vi "Main.vi"(11 "Module Admin":refnum<class "Delacor_lib_QMH_Module Admin.lvclass">) -> ()   [LabVIEW 2020, in "Display.lvlib"]
doc: "This template is based off of the Queued Message Handler design pattern and the Queued Message Handler project template that ships with LabVIEW.\n\nThe main difference is that the queue is private to this module and communication between modules is performed via Broadcast and Request events.\n\nRequest events are wrapped in public API methods and are handled in the Event Handling Loop (EHL) of this VI. Any module can register for Broadcast events sent by this module. The EHL generates messages based on user interface actions.\n\nThe Message Handling Loop (MHL) processes messages generated by the EHL, or by other messages. The messages are string values, so new messages can be added easily to the Message Cases case structure in the MHL. Each message cluster can also provide an optional value for Message Data, which is a variant that can be converted to whatever message-specific data is required.\n_____\nBased on Delacor QMH Project Template 5.0.0.82."
uses:
  Display.lvlib
  <vilib>/Delacor/Delacor QMH/Libraries/Module Admin_class/Delacor_lib_QMH_Module Admin.lvclass
  Module Data--cluster.ctl
  <vilib>/Delacor/Delacor QMH/Libraries/Message Queue_class/Delacor_lib_QMH_Message Queue.lvclass/Delacor_lib_QMH_Message Queue.ctl
  Stop Argument--cluster.ctl
  <vilib>/Delacor/Delacor QMH/Libraries/Module Admin_class/Delacor_lib_QMH_Module Admin.lvclass/Delacor_lib_QMH_Module Admin.ctl
  Simulation Argument--cluster.ctl
  <vilib>/Utility/miscctls.llb/LVPointTypeDef.ctl
  <vilib>/Delacor/Delacor QMH/Libraries/Message Queue_class/Delacor_lib_QMH_Enqueue Message (Single).vi
  <vilib>/Delacor/Delacor QMH/Libraries/Module Admin_class/Delacor_lib_QMH_Get External Launch.vi
  <vilib>/Utility/error.llb/Error Cluster From Error Code.vi
  <vilib>/ErrorRing/Error Ring.xnode
  <vilib>/Delacor/Delacor QMH/Libraries/Message Queue_class/Delacor_lib_QMH_Message Queue.lvclass
panel:
  out "ModuleName":string
  out "Sim?":bool
  in  "ExitMod":bool
  in  "Simulate MHL Error":bool
  in  "Simulate EHL Error":bool
  out "error out":errorcluster
  out "Status":string
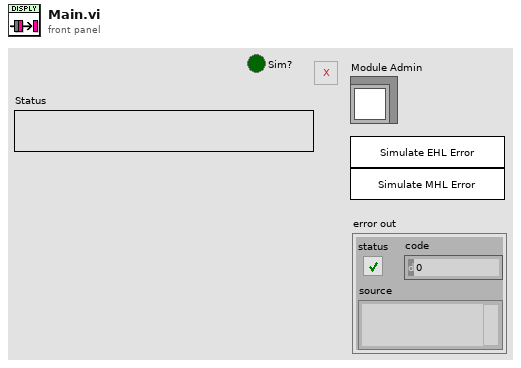
[diagram p1: front panel]
types:
  T1 = typedef "Display.lvlib/Request Events--cluster.ctl" = cluster{"Stop Module":refnum<user-event>, "Show Panel":refnum<user-event>, "Hide Panel":refnum<user-event>, "Get Module Execution Status":refnum<user-event>, "Show Diagram":refnum<user-event>, "Simulation":refnum<user-event>}
  T2 = typedef "Display.lvlib/Module Data--cluster.ctl" = cluster{"Status":string, "Sim":bool}
  T3 = enum32{"invalid lock state", "Not Locked", "Locked (No Password)", "Password-protected"}
  T4 = typedef "Display.lvlib/Stop Argument--cluster.ctl" = cluster{"Origin":string, "Exit via Stop Module Req?":bool, "Wait for Module to stop?":bool}
  T5 = typedef "Display.lvlib/Simulation Argument--cluster.ctl" = cluster{"Sim?":bool}
  T6 = typedef "LVPointTypeDef.ctl" = cluster{"Horizontal":i16, "Vertical":i16}
  T7 = enum32{"Invalid", "Standard", "Closed", "Hidden", "Minimized", "Maximized"}
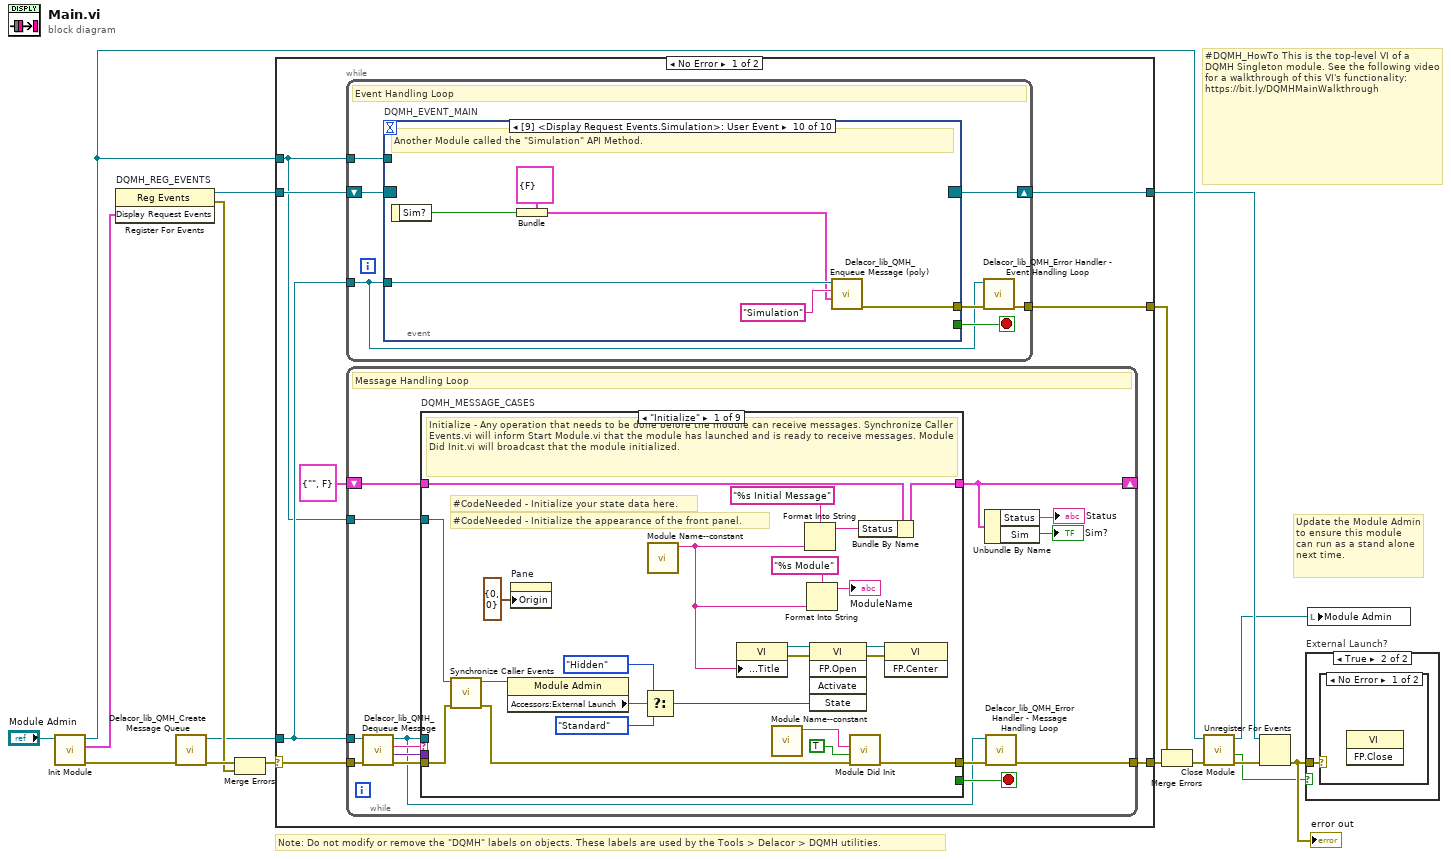
[diagram p0: block diagram]
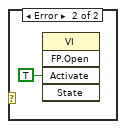
[diagram p3: hidden frame]
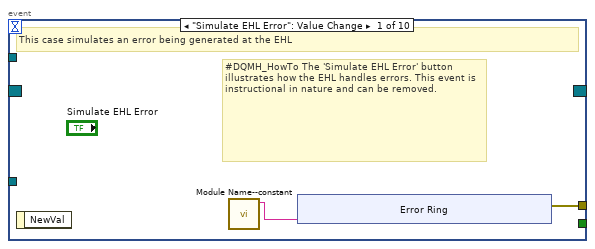
[diagram p4: hidden frame]
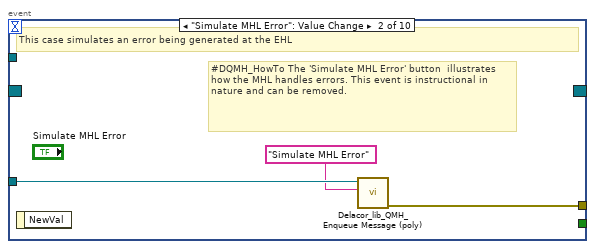
[diagram p5: hidden frame]
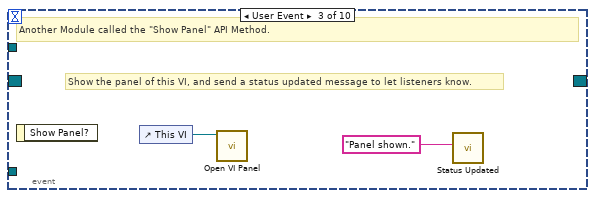
[diagram p6: hidden frame]
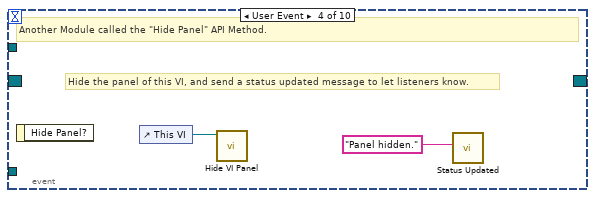
[diagram p7: hidden frame]
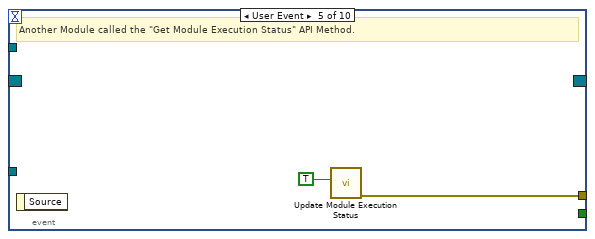
[diagram p8: hidden frame]
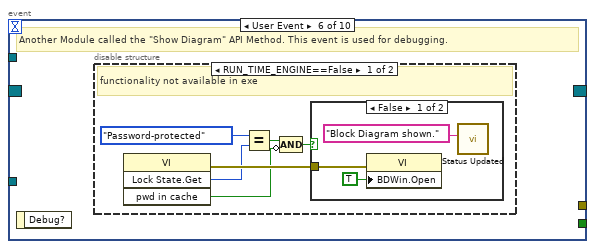
[diagram p9: hidden frame]
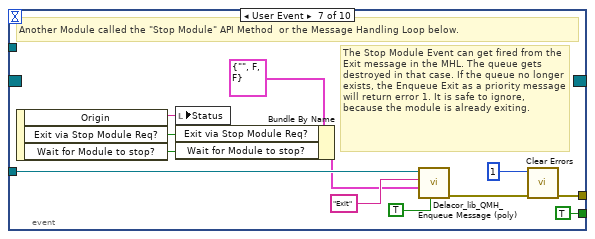
[diagram p12: hidden frame]
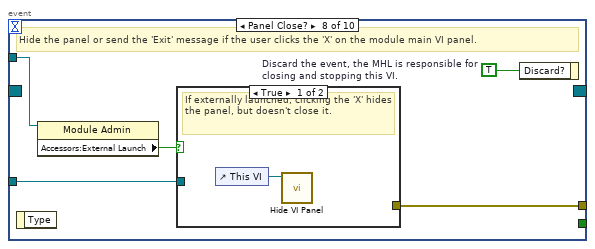
[diagram p13: hidden frame]
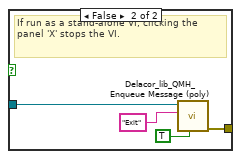
[diagram p14: hidden frame]
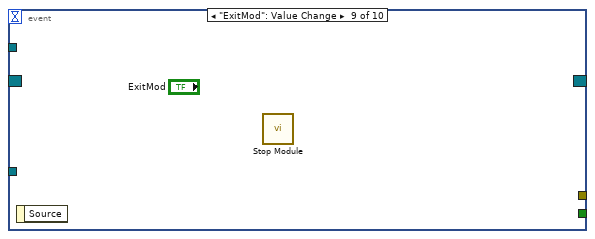
[diagram p15: hidden frame]
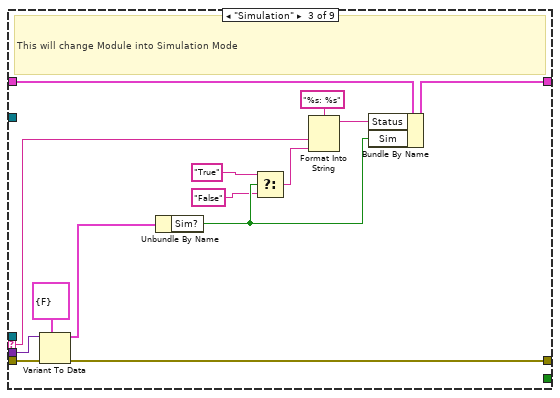
[diagram p17: hidden frame]
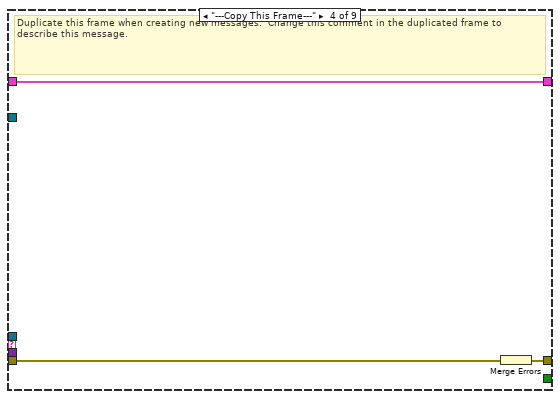
[diagram p18: hidden frame]
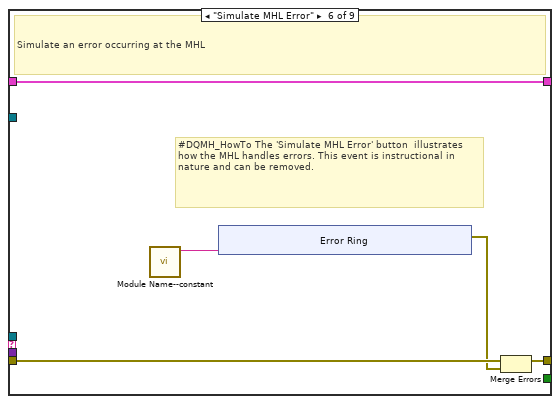
[diagram p20: hidden frame]
diagram:
  # "#DQMH_HowTo This is the top-level VI of a DQMH Singleton module. See the following video for a walkthrough of this VI's functionality: https://bit.ly/DQMHMainWalkthrough"
  # "Note: Do not modify or remove the \"DQMH\" labels on objects. These labels are used by the Tools > Delacor > DQMH utilities."
  # "Update the Module Admin to ensure this module can run as a stand alone next time."
  n1 = call "Init Module.vi"("Singleton Module Admin in"="Module Admin") -> ("error out"=w16:errorcluster, "Display Request Events"=w5:T1, "Singleton Module Admin out"=w8:refnum<class "Delacor_lib_QMH_Module Admin.lvclass">)  [unwired: 8 in]
  n2 = register-events "DQMH_REG_EVENTS"(w5) -> (reference out=w6:refnum<event-registration>, error out=w9:errorcluster)  [unwired: 2 in]
  n3 = call <vilib>:"Delacor_lib_QMH_Create Message Queue.vi"("error in"=w16) -> ("error out"=w11:errorcluster, "Message Queue"=w4:refnum<class "Delacor_lib_QMH_Message Queue.lvclass">)  [unwired: 9 in]
  n4 = Merge Errors(w11, w9) -> (w10:errorcluster)
  n5 = case shown="No Error" w10 {
    selector: w10 -> [w23 w206]
    tunnel: [w25 w205] -> w17
    tunnel: [w22 w211] -> w7
    tunnel: w6 -> [w20 w211]
    tunnel: w4 -> [w19 w204]
    tunnel: [w24 _] -> w14
    tunnel: w8 -> [w18 w207]
    frame No Error {
      n6 = while {
        tunnel: w19 -> [w26]
        shift-right: [w29] -> w22
        shift-left: w20 -> [w30]
        tunnel: [w31] -> w24
        tunnel: w18 -> [w27]
        stop <- w28 stop-if-true
        # "Event Handling Loop"
        n7 = event "DQMH_EVENT_MAIN" shown="[9] <Display Request Events.Simulation>: User Event" {
          selector: w30 -> [_ _ _ _ _ _ _ _ _ _]
          dyn-events: [_ _ _ _ _ _ _ _ _ _] -> w29
          timeout: _ -> [_ _ _ _ _ _ _ _ _ _]
          tunnel: [_ _ _ _ _ _ TRUE ("Discard?") _ _ _] -> w28
          tunnel: w26 -> [_ w43 _ _ _ _ w67 w74 _ w87]
          tunnel: [w34 w44 _ _ w50 _ w70 w76 _ w82] -> w32
          tunnel: w27 -> [_ _ _ _ _ _ _ w73 _ _]
          event "Simulate EHL Error": Value Change {
            # "#DQMH_HowTo The 'Simulate EHL Error' button  illustrates how the EHL handles errors. This event is instructional in nature and can be removed."
            # "This case simulates an error being generated at the EHL"
            n8 = event-data() -> ()  [unwired: 1 in, 1 out]
            n9 = call "Module Name--constant.vi"() -> ("Module Name"=w33:string)  [unwired: 11 in]
            n10 = xnode "Error Ring"("parameter 0"=w33) -> ("error out"=w34:errorcluster)
          }
          event "Simulate MHL Error": Value Change {
            # "#DQMH_HowTo The 'Simulate MHL Error' button  illustrates how the MHL handles errors. This event is instructional in nature and can be removed."
            # "This case simulates an error being generated at the EHL"
            n11 = event-data() -> ()  [unwired: 1 in, 1 out]
            n12 = call-poly <vilib>:"Delacor_lib_QMH_Enqueue Message (poly).vi"("Message"="Simulate MHL Error", "Message Queue in"=w43) -> ("error out"=w44:errorcluster)  [unwired: 8 in, 1 out]
          }
          event User Event {
            # "Show the panel of this VI, and send a status updated message to let listeners know."
            # "Another Module called the \"Show Panel\" API Method."
            n13 = event-data() -> ()  [unwired: 1 in, 1 out]
            n14 = control-ref of="This VI"() -> (w46:refnum<vi>)
            n15 = call "Open VI Panel.vi"("VI"=w46) -> ()  [unwired: 10 in, 1 out]
            n16 = call "Status Updated.vi"("Status"="Panel shown." ("format string")) -> ()  [unwired: 10 in, 1 out]
          }
          event User Event {
            # "Hide the panel of this VI, and send a status updated message to let listeners know."
            # "Another Module called the \"Hide Panel\" API Method."
            n17 = event-data() -> ()  [unwired: 1 in, 1 out]
            n18 = control-ref of="This VI"() -> (w48:refnum<vi>)
            n19 = call "Hide VI Panel.vi"("VI"=w48) -> ()  [unwired: 10 in, 1 out]
            n20 = call "Status Updated.vi"("Status"="Panel hidden." ("format string")) -> ()  [unwired: 10 in, 1 out]
          }
          event User Event {
            # "Another Module called the \"Get Module Execution Status\" API Method."
            n21 = event-data() -> ()  [unwired: 1 in, 1 out]
            n22 = call "Update Module Execution Status.vi"("Running?"=TRUE) -> ("error out"=w50:errorcluster)  [unwired: 10 in]
          }
          event User Event {
            # "Another Module called the \"Show Diagram\" API Method. This event is used for debugging."
            n23 = event-data() -> ()  [unwired: 1 in, 1 out]
            n24 = disable-structure shown="RUN_TIME_ENGINE==False" {
              frame condition #0 (active) {
                # "functionality not available in exe"
                n25 = invoke class="VI" method="Lock State.Get"() -> (error out=w56:errorcluster, "Get Lock State"=w55:T3, "pwd in cache"=w52:bool)  [unwired: 4 in, 1 out]
                n26 = Equal?(x=T3."Password-protected", y=w55) -> (x = y?=w53:bool)
                n27 = Compound Arithmetic op=AND(w53, invert w52) -> (w51:bool)
                n28 = case shown="False" w51 {
                  tunnel: w56 -> [w59 _]
                  frame False {
                    n29 = property class="VI"(error in=w59, "BDWin.Open"=TRUE ("Block Diagram Window:Open")) -> ()  [unwired: 1 in, 2 out]
                    n30 = call "Status Updated.vi"("Status"="Block Diagram shown." ("format string")) -> ()  [unwired: 10 in, 1 out]
                  }
                  frame True {
                    # "Password-protected VI, and the password is not in the cache. Do not show the diagram."
                  }
                }
              }
              frame condition #1 {
              }
            }
          }
          event User Event {
            # "The Stop Module Event can get fired from the Exit message in the MHL. The queue gets destroyed in that case. If the queue no longer exists, the Enqueue Exit as a priority message will return error 1. It is safe to ignore, because the module is already exiting."
            # "Another Module called the \"Stop Module\" API Method  or the Message Handling Loop below."
            n31 = event-data() -> ("Origin"=w66:string, "Exit via Stop Module Req?"=w62:bool, "Wait for Module to stop?"=w61:bool)  [unwired: 1 in]
            n32 = local write "Status"(w66) -> ()
            n33 = Bundle By Name(cluster=T4 {"Origin"="", "Exit via Stop Module Req?"=FALSE, "Wait for Module to stop?"=FALSE} ("Stop Argument"), "Exit via Stop Module Req?"=w62, "Wait for Module to stop?"=w61) -> (w60:T4)
            n34 = call-poly <vilib>:"Delacor_lib_QMH_Enqueue Message (poly).vi"("Priority Message? (F)"=TRUE, "Message Data"=w60, "Message"="Exit", "Message Queue in"=w67) -> ("error out"=w71:errorcluster)  [unwired: 6 in, 1 out]
            n35 = call <vilib>:"Clear Errors.vi"("error in (no error)"=w71, "specific error code to clear (0: all)"=1) -> ("error out"=w70:errorcluster)  [unwired: 4 in, 1 out]
          }
          event Panel Close? {
            w75 = TRUE  # Discard the event, the MHL is responsible for closing and stopping this VI.
            # "Hide the panel or send the 'Exit' message if the user clicks the 'X' on the module main VI panel."
            n36 = event-data() -> ()  [unwired: 1 in, 1 out]
            n37 = property class="Module Admin"(reference=w73) -> ("Accessors:External Launch"=w72:bool)  [unwired: 1 in, 2 out]
            n38 = case shown="True" w72 {
              tunnel: w74 -> [_ w80]
              tunnel: [_ w81] -> w76
              frame True {
                # "If externally launched, clicking the 'X' hides the panel, but doesn't close it."
                n39 = control-ref of="This VI"() -> (w77:refnum<vi>)
                n40 = call "Hide VI Panel.vi"("VI"=w77) -> ()  [unwired: 10 in, 1 out]
              }
              frame False {
                # "If run as a stand-alone VI, clicking the panel 'X' stops the VI."
                n41 = call-poly <vilib>:"Delacor_lib_QMH_Enqueue Message (poly).vi"("Priority Message? (F)"=TRUE, "Message"="Exit", "Message Queue in"=w80) -> ("error out"=w81:errorcluster)  [unwired: 7 in, 1 out]
              }
            }
            n42 = event-data("Discard?"=w75) -> ()  [unwired: 1 in, 1 out]
          }
          event "ExitMod": Value Change {
            n43 = event-data() -> ()  [unwired: 1 in, 1 out]
            n44 = call "Stop Module.vi"() -> ()  [unwired: 11 in, 1 out]
          }
          event User Event {
            # "Another Module called the \"Simulation\" API Method."
            n45 = event-data() -> ("Sim?"=w83:bool)  [unwired: 1 in]
            n46 = Bundle(cluster=T5 {"Sim?"=FALSE} ("Simulation Argument"), "Sim?"=w83) -> (w84:T5)
            n47 = call-poly <vilib>:"Delacor_lib_QMH_Enqueue Message (poly).vi"("Message Data"=w84, "Message"="Simulation", "Message Queue in"=w87) -> ("error out"=w82:errorcluster)  [unwired: 7 in, 1 out]
          }
        }
        n48 = call-dynamic "Delacor_lib_QMH_Error Handler - Event Handling Loop.vi"("error in"=w32, "Message Queue in"=w26) -> ("dup error in"=w31:errorcluster)  [unwired: 8 in, 1 out]
      }
      n49 = while {
        tunnel: w19 -> [w93]
        shift-right: [w90] -> _
        shift-left: T2 {"Status"="", "Sim"=FALSE} ("Data Cluster") -> [w97]
        tunnel: w23 -> [w100]
        tunnel: [w98] -> w25
        tunnel: w18 -> [w91]
        stop <- w96 stop-if-true
        # "Message Handling Loop"
        n50 = call-dynamic "Delacor_lib_QMH_Dequeue Message.vi"("error in"=w100, "Message Queue in"=w93) -> ("error out"=w99:errorcluster, "Message Data"=w94:variant, "Message"=w95:string, "Message Queue out"=w92:refnum<class "Delacor_lib_QMH_Message Queue.lvclass">)  [unwired: 6 in]
        n51 = case "DQMH_MESSAGE_CASES" shown="\"Initialize\"" w95 {
          selector: w95 -> [_ _ w133 _ _ _ _ _ w191]
          tunnel: w92 -> [_ _ _ _ _ _ w161 w183 _]
          tunnel: w99 -> [w122 w126 w140 w143 w145 w150 w168 w189 w193]
          tunnel: [w120 w126 w138 w142 w145 w149 w164 w186 w194] -> w101
          tunnel: w97 -> [w112 w125 w139 w141 w144 w147 w163 w182 w192]
          tunnel: [w111 w125 w134 w141 w144 w147 w163 w182 w192] -> w90
          tunnel: [_ _ _ _ _ _ _ w181 _] -> w96
          tunnel: w94 -> [_ _ w137 _ _ _ w162 w180 _]
          tunnel: w91 -> [w113 _ _ _ _ _ w160 w175 _]
          frame "Initialize" {
            # "#CodeNeeded - Initialize the appearance of the front panel."
            # "#CodeNeeded - Initialize your state data here."
            # "Initialize - Any operation that needs to be done before the module can receive messages. Synchronize Caller Events.vi will inform Start Module.vi that the module has launched and is ready to receive messages. Module Did Init.vi will broadcast that the module initialized."
            n52 = call "Synchronize Caller Events.vi"("error in (no error)"=w122, "Singleton Module Admin in"=w113) -> ("error out"=w121:errorcluster, "Singleton Module Admin out"=w108:refnum<class "Delacor_lib_QMH_Module Admin.lvclass">)  [unwired: 8 in]
            n53 = property class="Module Admin"(reference=w108) -> ("Accessors:External Launch"=w117:bool)  [unwired: 1 in, 2 out]
            n54 = property on="Pane" class="Pane"("Origin"=T6 {"Horizontal"=0, "Vertical"=0}) -> ()  [unwired: 2 in, 2 out]
            n55 = Select(t=T7."Hidden" ("State"), s=w117, f=T7."Standard" ("State")) -> (s? t:f=w114:T7)
            n56 = call "Module Name--constant.vi"() -> ("Module Name"=w104:string)  [unwired: 11 in]
            n57 = property class="VI"("Front Panel.Title"=w104) -> (reference out=w119:refnum<vi>, error out=w124:errorcluster)  [unwired: 2 in]
            n58 = call "Module Name--constant.vi"() -> ("Module Name"=w109:string)  [unwired: 11 in]
            n59 = Format Into String(format string="%s Initial Message" ("Initial Message"), w104) -> (resulting string=w106:string)  [unwired: 2 in, 1 out]
            n60 = Format Into String(format string="%s Module", w104) -> (resulting string=→"ModuleName":string)  [unwired: 2 in, 1 out]
            n61 = invoke class="VI" method="FP.Open"(reference=w119, error in=w124, "State"=w114) -> (reference out=w118:refnum<vi>, error out=w123:errorcluster)  [unwired: 2 in, 3 out]
            n62 = call "Module Did Init.vi"("error in (no error)"=w121, "Initialized?"=TRUE, "Origin"=w109) -> ("error out"=w120:errorcluster)  [unwired: 8 in]
            n63 = Bundle By Name(cluster=w112, "Status"=w106) -> (w111:T2)
            n64 = invoke class="VI" method="FP.Center"(reference=w118, error in=w123) -> ()  [unwired: 1 in, 3 out]
          }
          frame "--- Module Specific ---" {
            # "Separator -- The following cases handle messages specific to this Module."
          }
          frame "Simulation" {
            # "This will change Module into Simulation Mode"
            n65 = Variant To Data(error in=w140, type=T5 {"Sim?"=FALSE} ("Simulation Argument"), Variant=w137) -> (data=w135:T5, error out=w138:errorcluster)
            n66 = Unbundle By Name(w135) -> ("Sim?"=w132:bool)
            n67 = Select(t="True", s=w132, f="False") -> (s? t:f=w128:string)
            n68 = Format Into String(format string="%s: %s", w133, w128) -> (resulting string=w127:string)  [unwired: 2 in, 1 out]
            n69 = Bundle By Name(cluster=w139, "Status"=w127, "Sim"=w132) -> (w134:T2)
          }
          frame "---Copy This Frame---" {
            # "Duplicate this frame when creating new messages.  Change this comment in the duplicated frame to describe this message."
            n70 = Merge Errors(w143) -> (w142:errorcluster)
          }
          frame "--- Exit and Error Handling---" {
            # "Separator - The following cases handle errors and exit messages."
          }
          frame "Simulate MHL Error" {
            # "#DQMH_HowTo The 'Simulate MHL Error' button  illustrates how the MHL handles errors. This event is instructional in nature and can be removed."
            # "Simulate an error occurring at the MHL"
            n71 = call "Module Name--constant.vi"() -> ("Module Name"=w146:string)  [unwired: 11 in]
            n72 = xnode "Error Ring"("parameter 0"=w146) -> ("error out"=w148:errorcluster)
            n73 = Merge Errors(w150, w148) -> (w149:errorcluster)
          }
          frame "Error" {
            # "#CodeRecommended - If you ever change the name of this \"Error\" message, you'll need to update the name in the Check Loop Error.vi as well."
            # "#CodeRecommended - If the module is running in standalone mode (External Launch = FALSE), this code will pop up an error dialog and call the 'Exit' message if an error occurs. Add more fine-grained error handling here."
            # "Error - Check the error message data and respond accordingly. This message is sent by the \"Error Handler\" VIs at the end of each loop in this application."
            n74 = property class="Module Admin"(reference=w160) -> ("Accessors:External Launch"=w159:bool)  [unwired: 1 in, 2 out]
            n75 = Variant To Data(error in=w168, type=errorcluster {"status"=FALSE, "code"=0, "source"=""} ("error constant"), Variant=w162) -> (data=w169:errorcluster, error out=w166:errorcluster)
            n76 = call "Module Name--constant.vi"() -> ("Module Name"=w158:string)  [unwired: 11 in]
            n77 = call "Error Reported.vi"("Additional Information"=w158, "Error"=w169) -> ()  [unwired: 9 in, 1 out]
            n78 = case shown="False" w159 {
              tunnel: [w174 _] -> w165
              tunnel: w161 -> [w172 _]
              tunnel: w169 -> [w173 _]
              frame False {
                # "If the module is running standalone, then pop up an error dialog and call the \"Exit\" message."
                n79 = call <vilib>:"Simple Error Handler.vi"("error in (no error)"=w173) -> ()  [unwired: 4 in, 5 out]
                n80 = call-poly <vilib>:"Delacor_lib_QMH_Enqueue Message (poly).vi"("Priority Message? (F)"=TRUE, "Message"="Exit", "Message Queue in"=w172) -> ("error out"=w174:errorcluster)  [unwired: 7 in, 1 out]
              }
              frame True {
                # "If the module was launched externally, calling the Error Reported broadcast VI is the only action performed by the \"Error\" message. The module's caller can then process the error appropriately."
              }
            }
            n81 = Merge Errors(w166, w165) -> (w164:errorcluster)
            n82 = local write "error out"(w164) -> ()
          }
          frame "Exit" {
            w179 = 91  # 91: not all Exit messages will have an argument
            w181 = TRUE  # Stop the VI
            # "Release the message queue reference"
            # "#CodeNeeded - Add any required cleanup code here"
            # "Exit - Exit the application."
            n83 = Variant To Data(error in=w189, type=T4 {"Origin"="", "Exit via Stop Module Req?"=FALSE, "Wait for Module to stop?"=FALSE} ("Stop Argument"), Variant=w180) -> (data=w177:T4, error out=w185:errorcluster)
            n84 = call <vilib>:"Clear Errors.vi"("error in (no error)"=w185, "specific error code to clear (0: all)"=w179) -> ("error out"=w188:errorcluster)  [unwired: 4 in, 1 out]
            n85 = control-ref of="This VI"() -> (w176:refnum<vi>)
            n86 = call-dynamic "Delacor_lib_QMH_Release Message Queue.vi"("error in"=w188, "Message Queue"=w183) -> ("error out"=w187:errorcluster)  [unwired: 9 in]
            n87 = call "Handle Exit.vi"("Stop Argument"=w177, "Admin in"=w175, "VI reference"=w176) -> ("error out"=w184:errorcluster)  [unwired: 7 in, 1 out]
            n88 = Merge Errors(w187, w184) -> (w186:errorcluster)
          }
          frame Default {
            # "'Default' case only runs if there is a message that isn't defined in any of the other cases.  Output a programming error."
            n89 = call "Module Name--constant.vi"() -> ("Module Name"=w190:string)  [unwired: 11 in]
            n90 = xnode "Error Ring"("parameter 0"=w191, "parameter 1"=w190) -> ("error out"=w195:errorcluster)
            n91 = Merge Errors(w193, w195) -> (w194:errorcluster)
          }
        }
        n92 = Unbundle By Name(w90) -> ("Status"=→"Status":string, "Sim"=→"Sim?":bool)
        n93 = call-dynamic "Delacor_lib_QMH_Error Handler - Message Handling Loop.vi"("error in"=w101, "Message Queue in"=w92) -> ("dup error in"=w98:errorcluster)  [unwired: 8 in, 1 out]
      }
    }
    frame Error {
      # "Synchronize Caller Events.vi will inform Start Module.vi that the module has launched and will let the code calling Start Module.vi register for broadcasts and would permit the caller receive the broadcast that an error occurred at launch time."
      n94 = call-dynamic "Delacor_lib_QMH_Release Message Queue.vi"("error in"=w206, "Message Queue"=w204) -> ("error out"=w205:errorcluster)  [unwired: 9 in]
      n95 = call "Synchronize Caller Events.vi"("Singleton Module Admin in"=w207) -> ("error out"=w212:errorcluster)  [unwired: 9 in, 1 out]
      n96 = call "Module Name--constant.vi"() -> ("Module Name"=w210:string)  [unwired: 11 in]
      n97 = Format Into String(format string="An error occurred during initialization. %s is no longer running.", w210) -> (resulting string=w208:string)  [unwired: 2 in, 1 out]
      n98 = Merge Errors(w205, w212) -> (w213:errorcluster)
      n99 = call "Error Reported.vi"("Additional Information"=w208, "Error"=w213) -> ()  [unwired: 9 in, 1 out]
    }
  }
  n100 = Merge Errors(w14, w17) -> (w13:errorcluster)
  n101 = call "Close Module.vi"("error in (no error)"=w13, "Module Admin in"=w8) -> ("error out"=w15:errorcluster, "External Launch"=w1:bool, "Module Admin out"=w2:refnum<class "Delacor_lib_QMH_Module Admin.lvclass">)  [unwired: 7 in]
  n102 = Unregister For Events(event registration refnum=w7, error in=w15) -> (error out=w12:errorcluster)
  "error out" <- w12
  n103 = case "External Launch?" shown="True" w1 {
    tunnel: w12 -> [_ w214]
    frame False {
    }
    frame True {
      n104 = case shown="No Error" w214 {
        frame No Error {
          n105 = invoke class="VI" method="FP.Close"() -> ()  [unwired: 3 in, 3 out]
        }
        frame Error {
          n106 = invoke class="VI" method="FP.Open"("Activate"=TRUE ("Activate?")) -> ()  [unwired: 4 in, 5 out]
        }
      }
    }
  }
  n107 = local write "Module Admin"(w2) -> ()
